vi "draw vert line.vi"(10 "InRange":bool, 11 "Refnum in":T1) -> (3 "Refnum out":T1)   [LabVIEW 2015]
uses:
  <vilib>/vision/Image Controls.llb/IMAQ Image.ctl
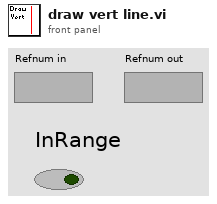
[diagram p1: front panel]
types:
  T1 = typedef "IMAQ Image.ctl" = refnum<image>
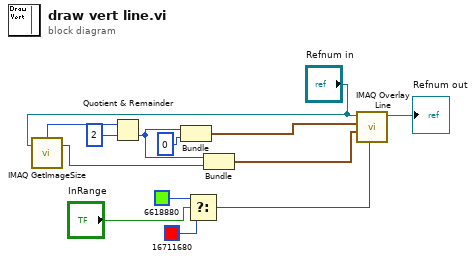
[diagram p0: block diagram]
diagram:
  n1 = call "IMAQ GetImageSize"("Image"="Refnum in") -> ("Y Resolution"=w12:i32, "X Resolution"=w6:i32)  [unwired: 3 in, 1 out]
  n2 = Quotient & Remainder(x=w6, y=2) -> (floor(x/y)=w9:i32)  [unwired: 1 out]
  n3 = Bundle(w9, "y"=0) -> (w8:cluster{i32, "y":i32})  [unwired: 1 in]
  n4 = Select(t=u32 6618880 ("Color"), s="InRange", f=u32 16711680 ("Color")) -> (s? t:f=w1:u32)
  n5 = Bundle(w9, "Y Resolution"=w12) -> (w10:cluster{i32, "Y Resolution":i32})  [unwired: 1 in]
  n6 = call "IMAQ Overlay Line"("Color"=w1, "End Point"=w10, "Start Point"=w8, "Image"="Refnum in") -> ("Image Out"=→"Refnum out":T1)  [unwired: 6 in, 1 out]
